vi "Set Subscribe Data.vi"(8 "error in (no error)":errorcluster, 9 "Message Transport Interface":refnum<class "Message Transport Interface.lvclass">, 10 "Subscriber Name":string, 11 "Topic Actor Subscribe Command in":refnum<class "Topic Actor Subscribe Command.lvclass">) -> (0 "error out":errorcluster, 3 "Topic Actor Subscribe Command out":refnum<class "Topic Actor Subscribe Command.lvclass">)   [LabVIEW 2016, in "Stream Mediator.lvlib" / "Topic Actor Subscribe Command.lvclass"]
doc: "--\nCopyright © 2017 Composed SystemsI All rights reserved.\n\nAuthor: Jon McBee <jon.mcbee@composed.io>\n\nThis library is provided \"AS IS\" ,WITHOUT WARRANTIES OR\nCONDITIONS OF ANY KIND, either express or implied.\n\nComposed Systems -- composed.io\n\nStream 0.0.1.1\nJon McBee - Composed Systems\nCopyright (c) 2017, Composed Systems"
uses:
  <userlib>/Composed Systems/Stream/Mediator/Classes/Topic Actor Subscribe Command/Topic Actor Subscribe Command.lvclass
  <userlib>/Composed Systems/Stream/Mediator/Classes/Message Transport Interface/Message Transport Interface.lvclass
  <userlib>/Composed Systems/Stream/Mediator/Classes/Topic Actor Subscribe Command/Topic Actor Subscribe Command.lvclass/Topic Actor Subscribe Command.ctl
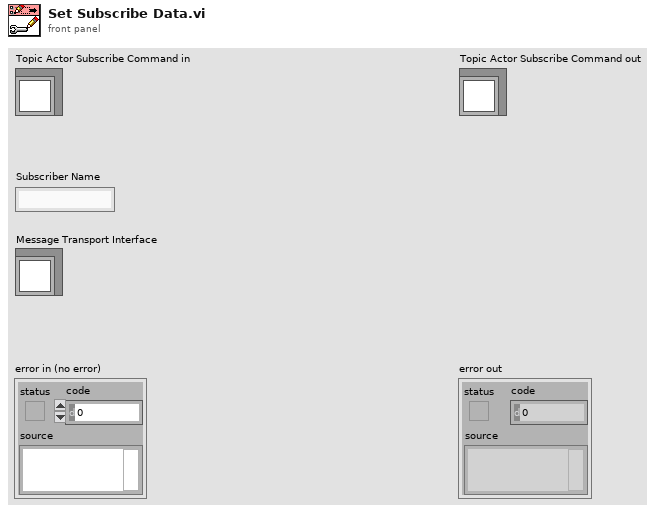
[diagram p1: front panel]
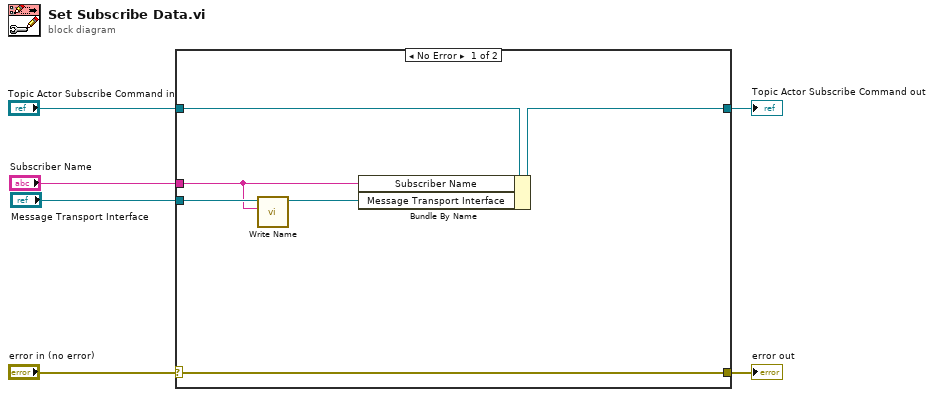
[diagram p0: block diagram]
diagram:
  n1 = case shown="No Error" "error in (no error)" {
    selector: "error in (no error)" -> [w12 w14]
    tunnel: [w12 w14] -> w5
    tunnel: [w10 w13] -> w3
    tunnel: "Topic Actor Subscribe Command in" -> [w11 w13]
    tunnel: "Subscriber Name" -> [w7 _]
    tunnel: "Message Transport Interface" -> [w9 _]
    frame No Error {
      n2 = call <userlib>:"Write Name.vi"("Name"=w7, "Message Transport Interface in"=w9) -> ("Message Transport Interface out"=w8:refnum<class "Message Transport Interface.lvclass">)  [unwired: 8 in, 1 out]
      n3 = Bundle By Name(cluster=w11, "Subscriber Name"=w7, "Message Transport Interface"=w8) -> (w10:refnum<class "Topic Actor Subscribe Command.lvclass">)
    }
    frame Error {
    }
  }
  "error out" <- w5
  "Topic Actor Subscribe Command out" <- w3
